vi "Configure Channel (DI Scale).vi"(0 "VISA resource name":refnum<visa-resource-name>, 1 "Scaling":T1={"Floating point position (2)"=2, "Lower Scaling (0)"=0.0, "Upper Scaling (100)"=100.0, "Unit Character (\"\")"=""} {"Upper Scaling (100)" format="%_6g"; "Lower Scaling (0)" format="%_6g"; "Floating point position (2)" min=0 max=5 step=1}, 5 "Channel (0001)":string="0001", 7 "Enable Channel (True)":bool=TRUE, 9 "Span":T2={"Lower Span (0)"=0, "Upper Span (1)"=1} {"Upper Span (1)" min=-99999 max=99999 step=1; "Lower Span (0)" min=-99999 max=99999 step=1}, 11 "error in (no error)":errorcluster) -> (4 "VISA resource name out":refnum<visa-resource-name>, 6 "Channel":string, 15 "error out":errorcluster)   [LabVIEW 2020, in "Yokogawa GX Series.lvlib"]
doc: "Sets the input range of DI channels.\n\nCommand: SRangeDI"
uses:
  <instrlib>/Yokogawa GX Series/Yokogawa GX Series.lvlib
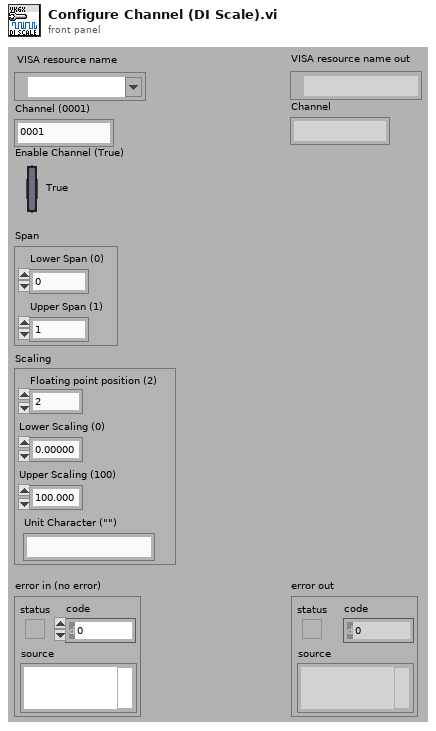
[diagram p1: front panel]
types:
  T1 = cluster{"Floating point position (2)":i32, "Lower Scaling (0)":dbl, "Upper Scaling (100)":dbl, "Unit Character (\"\")":string}
  T2 = cluster{"Lower Span (0)":i32, "Upper Span (1)":i32}
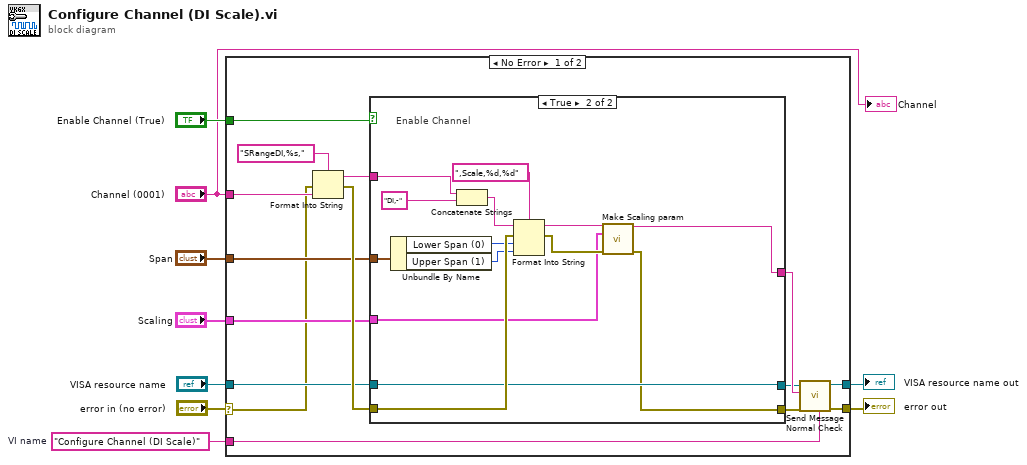
[diagram p0: block diagram]
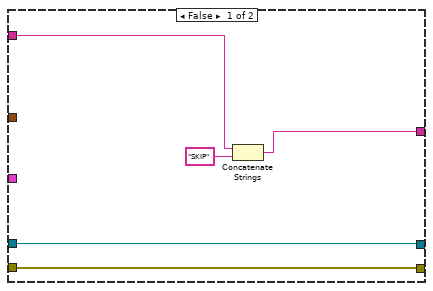
[diagram p2: hidden frame]
diagram:
  w7 = "Configure Channel (DI Scale)"  # VI name
  n1 = case shown="No Error" "error in (no error)" {
    selector: "error in (no error)" -> [w10 w44]
    tunnel: "Enable Channel (True)" -> [w21 _]
    tunnel: "Span" -> [w20 _]
    tunnel: w7 -> [w17 _]
    tunnel: [w16 w45] -> w6
    tunnel: [w15 w44] -> w5
    tunnel: "VISA resource name" -> [w13 w45]
    tunnel: "Scaling" -> [w12 _]
    tunnel: "Channel (0001)" -> [w11 _]
    frame No Error {
      n2 = Format Into String(format string="SRangeDI,%s,", error in=w10, w11) -> (resulting string=w22:string, error out=w23:errorcluster)  [unwired: 1 in]
      n3 = case shown="True" w21 {
        tunnel: w23 -> [w26 w42]
        tunnel: w22 -> [w27 w41]
        tunnel: [w26 w30] -> w19
        tunnel: [w28 w31] -> w18
        tunnel: w20 -> [_ w39]
        tunnel: [w25 w35] -> w14
        tunnel: w13 -> [w25 w35]
        tunnel: w12 -> [_ w32]
        frame False {
          n4 = Concatenate Strings(w27, "SKIP") -> (w28:string)
        }
        frame True {
          # "Enable Channel"
          n5 = Unbundle By Name(w39) -> ("Lower Span (0)"=w37:i32, "Upper Span (1)"=w36:i32)
          n6 = Concatenate Strings(w41, "DI,-") -> (w38:string)
          n7 = Format Into String(format string=",Scale,%d,%d", initial string=w38, error in=w42, w37, w36) -> (resulting string=w34:string, error out=w33:errorcluster)
          n8 = call <instrlib>:"Make Scaling param.vi"("String (\"\")"=w34, "Scaling"=w32, "error in (no error)"=w33) -> ("String After"=w31:string, "error out"=w30:errorcluster)  [unwired: 11 in]
        }
      }
      n9 = call <instrlib>:"Send Message Normal Check.vi"("Source (\"\")"=w17, "error in (no error)"=w19, "Send Message (\"\")"=w18, "VISA resource name"=w14) -> ("error out"=w15:errorcluster, "VISA resource name out"=w16:refnum<visa-resource-name>)  [unwired: 2 in, 4 out]
    }
    frame Error {
    }
  }
  "error out" <- w5
  "VISA resource name out" <- w6
  "Channel" <- "Channel (0001)"
